vi "Entity Definition.vi"(11 "Path":path) -> (0 "error out":errorcluster, 3 "Definition":refnum<class "Type.lvclass">[](array[class]), 5 "Result Types":string[](array[string]))   [LabVIEW 2020, in "Conditum-Tools.lvlib" / "Entity Editor.lvclass"]
uses:
  Entity Editor.lvclass
  Conditum-Clone/Columns/Type/Type.lvclass
  550162fa-cd4f-47e4-bfa0-f6c4a8cf26d7.vi
  faf18998-b64d-43fd-aea9-487060b028ef.vi
  Entity Definition OoC.vi
  Entity Editor.lvclass/Entity Editor.ctl
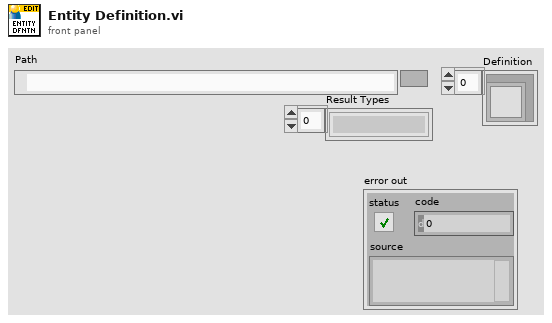
[diagram p1: front panel]
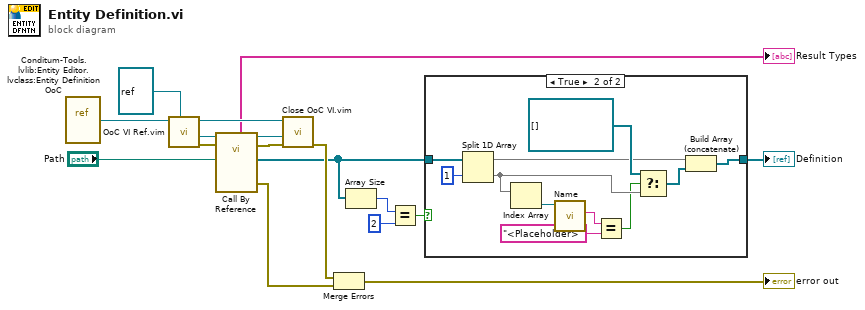
[diagram p0: block diagram]
diagram:
  n1 = vi-ref "Conditum-Tools.lvlib:Entity Editor.lvclass:Entity Definition OoC.vi"() -> (w12:refnum<vi>)
  n2 = call "OoC VI Ref.vim"("VI Type"=refnum<vi> refnum, "OoC SVR"=w12) -> ("error out"=w15:errorcluster, "vi reference"=w16:refnum<vi>, "context"=w14:refnum<vi>)  [unwired: 7 in]
  n3 = call-by-ref "?"(reference=w16, error in=w15, "Entity path"="Path") -> (reference out=w13:refnum<vi>, error out=w6:errorcluster, 0:"error out"=w9:errorcluster, "Definition"=w2:refnum<class "Type.lvclass">[], "Result Types"=→"Result Types":string[])  [unwired: 8 in]
  n4 = call "Close OoC VI.vim"("error in (no error)"=w6, "vi reference"=w13, "context"=w14) -> ("error out"=w17:errorcluster)  [unwired: 8 in]
  n5 = Merge Errors(w17, w9) -> (→"error out":errorcluster)
  n6 = Array Size(array=w2) -> (size(s)=w5:i32)
  n7 = Equal?(x=w5, y=2) -> (x = y?=w3:bool)
  n8 = case shown="True" w3 {
    tunnel: w2 -> [w18 w28]
    tunnel: [w18 w19] -> w1
    frame False {
    }
    frame True {
      n9 = Split 1D Array(array=w28, index=1) -> (first subarray=w21:refnum<class "Type.lvclass">[], second subarray=w24:refnum<class "Type.lvclass">[])
      n10 = Index Array(array=w24) -> (element=w25:refnum<class "Type.lvclass">)  [unwired: 1 in]
      n11 = call "Name.vi"("Type in"=w25) -> ("Table Name"=w27:string)  [unwired: 10 in]
      n12 = Equal?(x=w27, y="<Placeholder>") -> (x = y?=w22:bool)
      n13 = Select(t=refnum<class "Type.lvclass">[] [], s=w22, f=w24) -> (s? t:f=w20:refnum<class "Type.lvclass">[])
      n14 = Build Array (concatenate)(w21, w20) -> (w19:refnum<class "Type.lvclass">[])
    }
  }
  "Definition" <- w1
